vi "E816_Simple_Test.vi"() -> ()   [LabVIEW 2020]
doc: "This simple test VI is a stand-alone sample application. Use the \nHelp - Show Context Help menu sequence in the LabVIEW environment to display the Context Help window with the VI and control/indicator descriptions.\n\nSpecify first: \n¢ System no. (= 1 in a one-system configuration),\n¢ Interface (RS232 or USB),\n¢ For Interface = RS232: appropriate port number and RS232 baud rate. If you do not know the baud rate settings of the connected E-816, leave Try different baudrates? TRUE. The VI will then try to find the correct baudrate automatically by calling \"Find baudrate.vi\".\n¢ For Interface = USB: appropriate Serial Number of the controller to connect to or if you want to search for the controller.\n¢ Timeout value (im milliseconds)\n\nThen start the VI. The VI will open a connection to the E-816 and query the controller for the available axis IDs, position values of these axes, and the master E-816 identification string. The diagram shows how to combine the driver and support VIs for these tasks."
panel:
  in  "Wait":string="Please wait.\nChecking for correct baudrate."
  in  "Interface":u16(ring) items=["RS232", "USB"]
  in  "USB settings":cluster{"S/N":string, "USB Search?":bool}={"S/N"="", "USB Search?"=TRUE}
  in  "RS232 settings":cluster{"Portnumber":i32, "Baudrate":u16}={"Portnumber"=0, "Baudrate"=4} {"Portnumber" items=["COM1", "COM2", "COM3", "COM4", "COM5", "COM6", "COM7", "COM8", "COM9", "COM10", "COM11", "COM12", "COM13", "COM14", "COM15", "COM16", "COM17", "COM18", "COM19", "COM20", "COM21", "COM22", "COM23", "COM24", "COM25", "COM26", "COM27", "COM28", "COM29", "COM30"]; "Baudrate" items=["9600", "14400", "19200", "38400", "57600", "115200"]}
  in  "error in":errorcluster
  in  "System no.":i32=1 min=1 step=1
  in  "Try different baudrates?":bool=TRUE
  in  "Timeout":i32=5000
  out "error out":errorcluster
  out "Position":dbl[](array[numeric]) format="%.6f"
  out "Conn. Axes":string[](array[string])
  out "Identification":string="\n"
  # "Simple E-816 communication test program"
  # "Select Interface settings first, then start the VI. If Interface = RS232 and you\ndon't know the correct Baudrate, leave \"Try different baudrates?\" TRUE. If\nInterface = USB and you don't know the serial number, leave \"USB Search?\" = TRUE. Then start the VI. \nThe VI will open the chosen port, query for connected axes (SAI?), position (POS?), and master E-816\nIdentification (*IDN?). See VI and control/ indicator information for details."
  # "Only for\nInterface = \nRS232:"
  # "Only for\nInterface = \nUSB:"
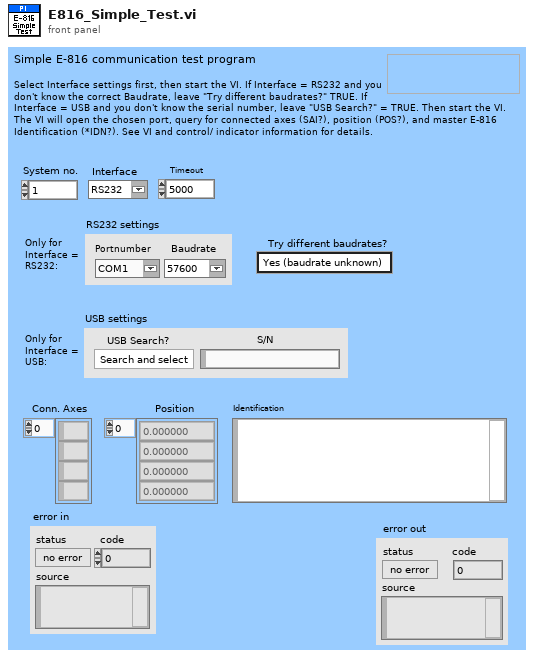
[diagram p1: front panel]
types:
  T1 = enum16{"DCO", "DCO?", "MOV", "MOV?", "MVR", "ONT?", "OVF?", "POS?", "RST", "SVA", "SVA?", "SVO", "SVO?", "SVR", "VOL?"}
  T2 = cluster{"input XON/XOFF":bool, "input HW Handshake":bool, "input alt HW HShk":bool, "output XON/XOFF":bool, "output HW Handshake":bool, "output alt HW HShk":bool, "XOFF byte":u8, "XON byte":u8, "parity error byte":u16}
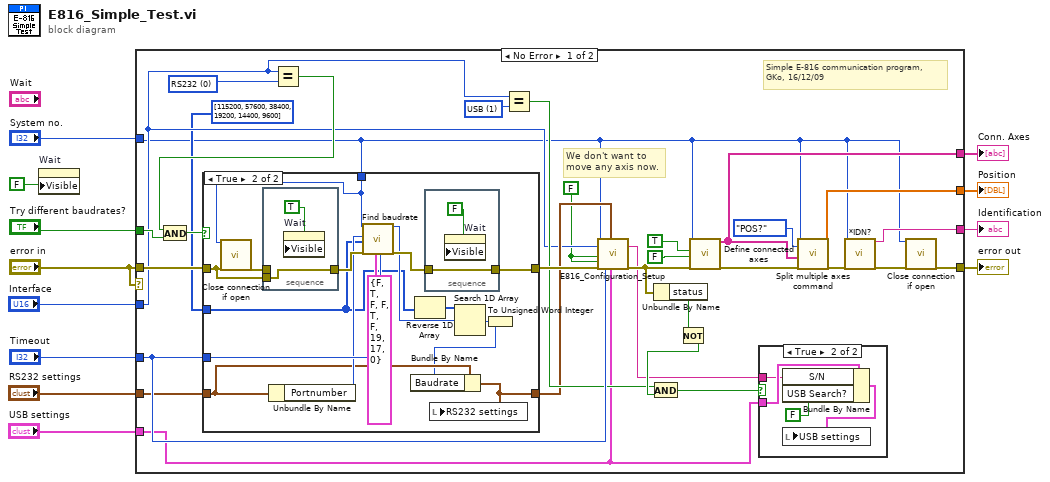
[diagram p0: block diagram]
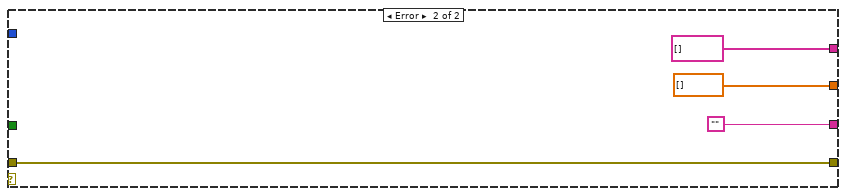
[diagram p4: hidden frame]
diagram:
  n1 = property on="Wait" class="Str"("Visible"=FALSE ("Write Attribute")) -> ()  [unwired: 2 in, 2 out]
  n2 = case shown="No Error" "error in" {
    tunnel: [w14 w73] -> w12
    tunnel: "error in" -> [w40 w73]
    tunnel: "System no." -> [w13 _]
    tunnel: "Try different baudrates?" -> [w26 _]
    tunnel: "Timeout" -> [w37 _]
    tunnel: [w36 "" ("Identification")] -> w6
    tunnel: [w35 dbl[] [] ("Num. values out")] -> w5
    tunnel: [w34 string[] [] ("Conn. Axes out")] -> w4
    tunnel: "Interface" -> [w18 _]
    tunnel: "USB settings" -> [w21 _]
    tunnel: "RS232 settings" -> [w20 _]
    frame No Error {
      w24 = u16 1 items=["RS232", "USB"] ("Interface")
      w25 = u16 0 items=["RS232", "USB"] ("Interface")
      w16 = FALSE ("Change servo \nstatus to ON?")
      # "We don't want to\nmove any axis now."
      # "Simple E-816 communication program,\nGKo, 16/12/09"
      n3 = Equal?(x=w18, y=w25) -> (x = y?=w27:bool)
      n4 = And(x=w27, y=w26) -> (x .and. y?=w28:bool)
      n5 = case shown="True" w28 {
        tunnel: [w49 w65] -> w39
        tunnel: w40 -> [w49 w50]
        tunnel: w37 -> [_ w62]
        tunnel: w13 -> [_ w53]
        tunnel: u32[] [115200, 57600, 38400, 19200, 14400, 9600] ("Valid Baudrates") -> [_ w52]
        tunnel: w20 -> [w48 w58]
        tunnel: [w48 w56] -> w19
        frame False {
        }
        frame True {
          n6 = call "Close connection if open.vi"("System no."=w53, "error in"=w50) -> ("error out"=w54:errorcluster)  [unwired: 1 in, 16 out]
          n7 = stacked-sequence {
            tunnel: w54 -> [_]
            tunnel: [w66] -> w63
            tunnel: w50 -> [w66]
            frame #0 {
              n8 = property on="Wait" class="Str"("Visible"=TRUE ("Write Attribute")) -> ()  [unwired: 2 in, 2 out]
            }
          }
          n9 = Unbundle By Name(w58) -> ("Portnumber"=w59:i32)
          n10 = call "Find baudrate.vi"("System no."=w53, "RS-232 Portnumber"=w59, "Valid Baudrates"=w52, "error in"=w63, "Flow control"=T2 {"input XON/XOFF"=FALSE, "input HW Handshake"=TRUE, "input alt HW HShk"=FALSE, "output XON/XOFF"=FALSE, "output HW Handshake"=TRUE, "output alt HW HShk"=FALSE, "XOFF byte"=19, "XON byte"=17, "parity error byte"=0}, "Timeout"=w62) -> ("Baudrate out"=w60:u32, "error out"=w64:errorcluster)  [unwired: 5 in, 7 out]
          n11 = Reverse 1D Array(array=w52) -> (reversed array=w51:u32[])
          n12 = stacked-sequence {
            tunnel: w64 -> [w68]
            tunnel: [w68] -> w65
            frame #0 {
              n13 = property on="Wait" class="Str"("Visible"=FALSE ("Write Attribute")) -> ()  [unwired: 2 in, 2 out]
            }
          }
          n14 = Search 1D Array(1D array=w51, element=w60) -> (index of element=w61:i32)  [unwired: 1 out]
          n15 = To Unsigned Word Integer(number=w61) -> (unsigned 16bit integer=w57:u16)
          n16 = Bundle By Name(cluster=w58, "Baudrate"=w57) -> (w56:cluster{"Portnumber":i32, "Baudrate":u16})
          n17 = local write "RS232 settings"(w56) -> ()
        }
      }
      n18 = Equal?(x=w18, y=w24) -> (x = y?=w23:bool)
      n19 = call "E816_Configuration_Setup.vi"("System no."=w13, "Interface"=w18, "All axes?"=w16, "Change servo \nstatus to ON?"=w16, "error in"=w39, "Timeout"=w37, "RS232 settings"=w19, "USB settings"=w21) -> ("SN out"=w22:string, "error out"=w30:errorcluster)  [unwired: 2 in, 8 out]
      n20 = Unbundle By Name(w30) -> ("status"=w29:bool)
      n21 = Not(x=w29) -> (.not. x?=w31:bool)
      n22 = And(x=w23, y=w31) -> (x .and. y?=w32:bool)
      n23 = call "Define connected axes.vi"("System no."=w13, "Read from\ncontroller?"=TRUE ("Read from\nController"), "Invert\norder?"=FALSE ("Invert\nOrder"), "error in"=w30) -> ("Conn. Axes out"=w34:string[], "error out"=w41:errorcluster)  [unwired: 1 in, 13 out]
      n24 = case shown="True" w32 {
        tunnel: w21 -> [_ w47]
        tunnel: w22 -> [_ w46]
        frame False {
        }
        frame True {
          n25 = Bundle By Name(cluster=w47, "S/N"=w46, "USB Search?"=FALSE) -> (w44:cluster{"S/N":string, "USB Search?":bool})
          n26 = local write "USB settings"(w44) -> ()
        }
      }
      n27 = call "Split multiple axes command.vi"("System no."=w13, "Command"=T1."POS?", "Axes to command"=w34, "error in"=w41) -> ("Num. values out"=w35:dbl[], "error out"=w38:errorcluster)  [unwired: 5 in, 9 out]
      n28 = call "*IDN?.vi"("System no."=w13, "error in"=w38) -> ("Identification"=w36:string, "error out"=w15:errorcluster)  [unwired: 16 out]
      n29 = call "Close connection if open.vi"("System no."=w13, "error in"=w15) -> ("error out"=w14:errorcluster)  [unwired: 1 in, 16 out]
    }
    frame Error {
    }
  }
  "error out" <- w12
  "Identification" <- w6
  "Position" <- w5
  "Conn. Axes" <- w4
